vi "Connect.vi"(6 "remote_port":u16, 7 "host_port":u16, 8 "error in (no error)":errorcluster, 9 "remote_address":string, 10 "host_address":string, 11 "Socket.UDP in":refnum<class "Socket.UDP.lvclass">) -> (0 "error out":errorcluster, 3 "Socket.UDP out":refnum<class "Socket.UDP.lvclass">)   [LabVIEW 2014, in "Socket.lvlib" / "Socket.UDP.lvclass"]
doc: "string host_address is the optional address of the host. Usage varies depending on the transfer_mode:\n point-to-point: host address becomes both the net address and the service name of the UDP connection. If left blank, the connection will use all Ethernet cards on the machine.\n multicast: host address will be used as the net address for the connection.\n broadcast: host address is not used but is stored in the properties for later use.\n \nu16 host_port is the optional port to connect to on the host. Usage varies depending on the transfer_mode:\n point-to-point: host_port is the connection port number.\n multicast: if host_port is 0, then the connection is write-only (server),, if host_port is not 0, then the connection is read-only (client) and host_port is the port that the connection will listen on.\n broadcast: if host port is 0, then the connection will be a server. If not 0, then the connection will be a client and host_port is the port that the client will listen on.\n\n string remote_address the address to connect to the remote target. Usage varies depending on the transfer_mode:\n point-to-point: not used by connection but stored in the properties for later use.\n multicast: if host_port is 0 then the connection is write only (server) and remote_address is not used by the connect method but stored in the properties for later use. If host_port is not 0, then the connection is read only (client) and the remote port is the port that the client will listen on.\n\nstring remote_port is the port to connect to on the remote target. Not used by the Connect method but saved in the properties for future use."
uses:
  Socket.UDP.lvclass
  Socket.UDP.lvclass/Socket.UDP.ctl
  Socket.Base/Socket.Base.lvclass/Socket.Base.ctl
  Accessors/Read transfer_mode.vi
  Socket.Base/Accessors/Read timeout.vi
  Accessors/Read time-to-live.vi
  Accessors/Write host_address.vi
  Accessors/Write host_port.vi
  Accessors/Write remote_address .vi
  Accessors/Write remote_port .vi
  Accessors/Write udp_refnum.vi
  Socket.Base/Accessors/Write connected.vi
  <vilib>/Utility/tcp.llb/UDP Multicast Read-Only Open.vi
  <vilib>/Utility/tcp.llb/UDP Multicast Write-Only Open.vi
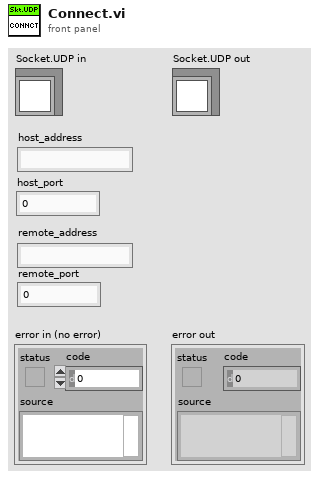
[diagram p1: front panel]
types:
  T1 = enum16{"point-to-point", "multicast", "broadcast"}
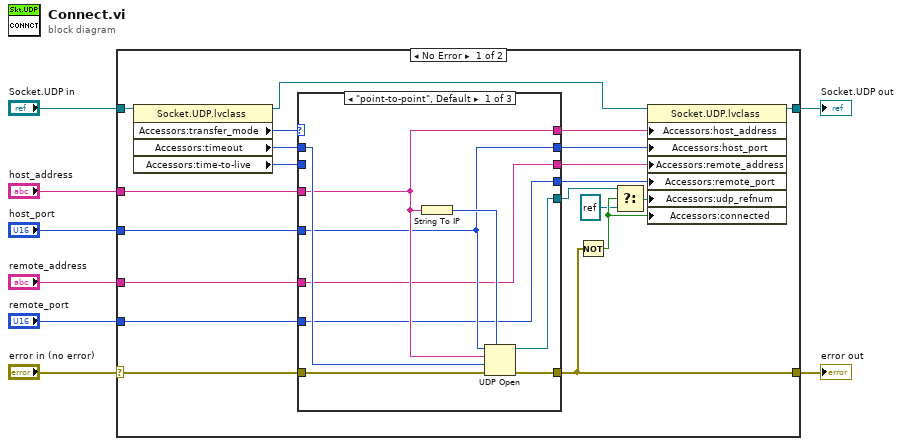
[diagram p0: block diagram]
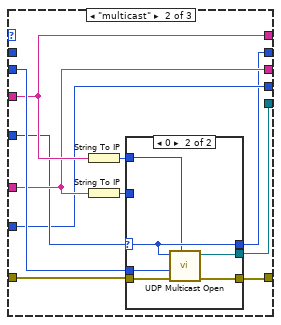
[diagram p2: hidden frame]
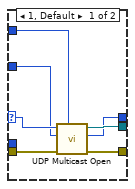
[diagram p3: hidden frame]
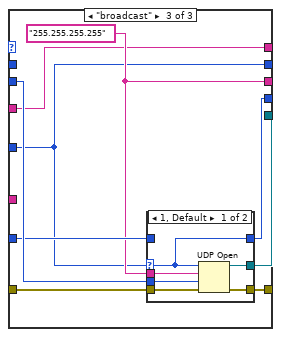
[diagram p4: hidden frame]
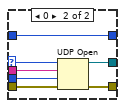
[diagram p5: hidden frame]
diagram:
  n1 = case shown="No Error" "error in (no error)" {
    selector: "error in (no error)" -> [w24 w85]
    tunnel: [w16 w85] -> w7
    tunnel: [w13 w84] -> w5
    tunnel: "Socket.UDP in" -> [w28 w84]
    tunnel: "host_address" -> [w25 _]
    tunnel: "host_port" -> [w23 _]
    tunnel: "remote_address" -> [w20 _]
    tunnel: "remote_port" -> [w17 _]
    frame No Error {
      n2 = property class="Socket.UDP.lvclass"(reference=w28) -> (reference out=w15:refnum<class "Socket.UDP.lvclass">, "Accessors:transfer_mode"=w27:T1, "Accessors:timeout"=w26:i32, "Accessors:time-to-live"=w14:u16)  [unwired: 1 in, 1 out]
      n3 = case shown="\"point-to-point\", Default" w27 {
        tunnel: w26 -> [w36 _ _]
        tunnel: w25 -> [w34 w44 w64]
        tunnel: w24 -> [w37 w47 w70]
        tunnel: w23 -> [w33 w42 w63]
        tunnel: [w34 w44 w64] -> w22
        tunnel: [w33 w39 w63] -> w21
        tunnel: w20 -> [w32 w43 _]
        tunnel: [w32 w43 w65] -> w19
        tunnel: [w31 w41 w62] -> w18
        tunnel: w17 -> [w31 w41 w66]
        tunnel: [w30 w40 w68] -> w11
        tunnel: [w29 w38 w69] -> w16
        tunnel: w14 -> [_ w48 w67]
        frame "point-to-point", Default {
          n4 = String To IP(1:w34) -> (0:w35:u32)
          n5 = UDP Open(7:w35, 8:w37, 9:w36, 10:w34, 11:w33) -> (port=w30:refnum<k16>, 0:w29:errorcluster)  [unwired: 1 out]
        }
        frame "multicast" {
          n6 = String To IP(1:w44) -> (0:w45:u32)
          n7 = String To IP(1:w43) -> (0:w46:u32)
          n8 = case shown="0" w42 {
            selector: w42 -> [w53 w59]
            tunnel: w47 -> [w55 w61]
            tunnel: w45 -> [w54 w56]
            tunnel: w46 -> [w52 _]
            tunnel: [w51 w58] -> w38
            tunnel: [w50 w60] -> w40
            tunnel: [w49 w59] -> w39
            tunnel: w48 -> [_ w57]
            frame 1, Default {
              n9 = call-poly <vilib>:"UDP Multicast Open.vi"("net address"=w54, "error in (no error)"=w55, "multicast addr"=w52, "port"=w53) -> ("error out"=w51:errorcluster, "port out"=w49:u16, "connection ID"=w50:refnum<k16>)  [unwired: 5 in]
            }
            frame 0 {
              n10 = call-poly <vilib>:"UDP Multicast Open.vi"("net address"=w56, "error in (no error)"=w61, "time-to-live (1)"=w57, "port"=w59) -> ("error out"=w58:errorcluster, "connection ID"=w60:refnum<k16>)  [unwired: 6 in]
            }
          }
        }
        frame "broadcast" {
          w65 = "255.255.255.255"
          n11 = case shown="1, Default" w63 {
            selector: w63 -> [w71 w78]
            tunnel: w67 -> [w76 w83]
            tunnel: w70 -> [w75 w82]
            tunnel: [w74 w81] -> w68
            tunnel: [w73 w80] -> w69
            tunnel: w66 -> [_ w77]
            tunnel: w65 -> [w72 w79]
            tunnel: [w71 w77] -> w62
            frame 1, Default {
              n12 = UDP Open(8:w75, 9:w76, 10:w72, 11:w71) -> (port=w74:refnum<k16>, 0:w73:errorcluster)  [unwired: 1 in, 1 out]
            }
            frame 0 {
              n13 = UDP Open(8:w82, 9:w83, 10:w79, 11:w78) -> (port=w81:refnum<k16>, 0:w80:errorcluster)  [unwired: 1 in, 1 out]
            }
          }
        }
      }
      n14 = Not(x=w16) -> (.not. x?=w10:bool)
      n15 = Select(t=w11, s=w10, f=refnum<k16> refnum) -> (s? t:f=w12:refnum<k16>)
      n16 = property class="Socket.UDP.lvclass"(reference=w15, "Accessors:host_address"=w22, "Accessors:host_port"=w21, "Accessors:remote_address "=w19, "Accessors:remote_port "=w18, "Accessors:udp_refnum"=w12, "Accessors:connected"=w10) -> (reference out=w13:refnum<class "Socket.UDP.lvclass">)  [unwired: 1 in, 1 out]
    }
    frame Error {
    }
  }
  "error out" <- w7
  "Socket.UDP out" <- w5
